vi "Pico1-1.vi"(7 "ajout test#":string, 11 "Datain":T1) -> (2 "taboutBdd":string[](array[string]), 3 "Chaîne":string)   [LabVIEW 2020]
panel:
  # "29/08/2022_09:32;Test# 5 - predcir;23.5000;23.5000;23.6000;23.6000;3.6304;3.6291;3.6291;3.6291;"
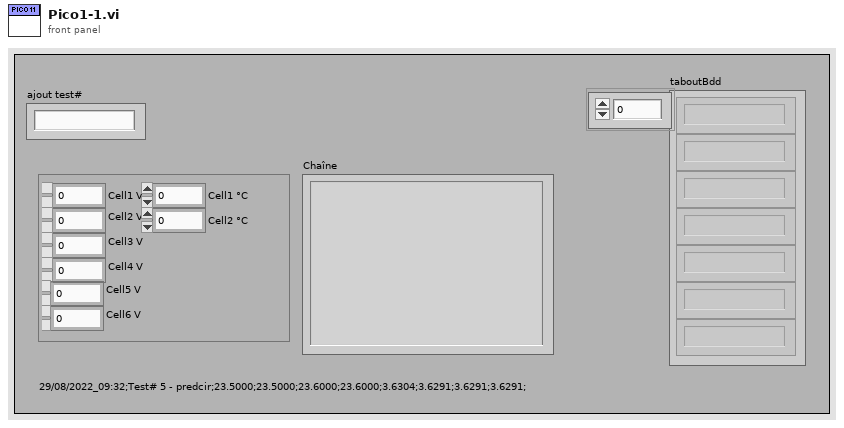
[diagram p1: front panel]
types:
  T1 = cluster{"Cell1 V":sgl, "Cell2 V":sgl, "Cell3 V":sgl, "Cell4 V":sgl, "Cell1 °C":sgl, "Cell2 °C":sgl, "Cell5 V":sgl, "Cell6 V":sgl}
  T2 = cluster{"Cell1 V":sgl, "Cell2 V":sgl, "Cell3 V":sgl, "Cell4 V":sgl, "Cell5 V":sgl, "Cell6 V":sgl, "Cell1 °C":sgl, "Cell2 °C":sgl}
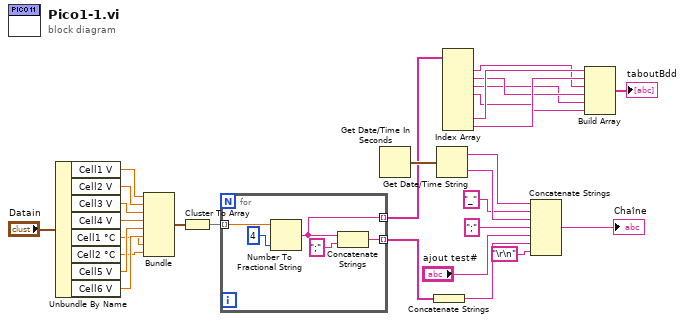
[diagram p0: block diagram]
diagram:
  n1 = Unbundle By Name("Datain") -> ("Cell1 V"=w15:sgl, "Cell2 V"=w14:sgl, "Cell3 V"=w13:sgl, "Cell4 V"=w12:sgl, "Cell1 °C"=w9:sgl, "Cell2 °C"=w8:sgl, "Cell5 V"=w11:sgl, "Cell6 V"=w10:sgl)
  n2 = Bundle("Cell1 V"=w15, "Cell2 V"=w14, "Cell3 V"=w13, "Cell4 V"=w12, "Cell5 V"=w11, "Cell6 V"=w10, "Cell1 °C"=w9, "Cell2 °C"=w8) -> (w7:T2)  [unwired: 1 in]
  n3 = Cluster To Array(cluster=w7) -> (array=w21:sgl[])
  n4 = for {
    tunnel: [w31] -> w18 mode=indexing
    tunnel: w21 -> [w33] mode=indexing
    tunnel: [w30] -> w17 mode=indexing
    n5 = Number To Fractional String(number=w33, precision (6)=i16 4 ("précision (6)")) -> (F-format string=w30:string)  [unwired: 2 in]
    n6 = Concatenate Strings(w30, ";" ("chaîne")) -> (w31:string)
  }
  n7 = Get Date/Time In Seconds() -> (seconds since 1Jan1904=w28:timestamp)
  n8 = Concatenate Strings(w18) -> (w23:string)
  n9 = Get Date/Time String(seconds (now)=w28) -> (date string=w27:string, time string=w26:string)  [unwired: 2 in]
  n10 = Index Array(array=w17) -> (element #1=w4:string, element #2=w3:string, element #3=w2:string, element #4=w1:string, element #7=w6:string, element #8=w5:string)  [unwired: 8 in, 2 out]
  n11 = Concatenate Strings(w27, "_" ("chaîne"), w26, ";" ("chaîne"), "ajout test#", w23, "\r\n") -> (→"Chaîne":string)
  n12 = Build Array(w6, w5, w4, w3, w2, w1) -> (→"taboutBdd":string[])
